vi "DecodeImageArray.vi"(5 "Height":i32, 6 "Pixel Format":T1, 7 "Width":i32, 8 "error in (no error)":errorcluster, 10 "Array":u8[](array[numeric]), 11 "image  in":T2) -> (0 "error out":errorcluster, 3 "image out":T2)   [LabVIEW 2021]
uses:
  <vilib>/vision/Image Controls.llb/IMAQ Image.ctl
  PixelFormat.ctl
  bayer_decode.ctl
panel:
  out "Raw Bytes Per frame":i32
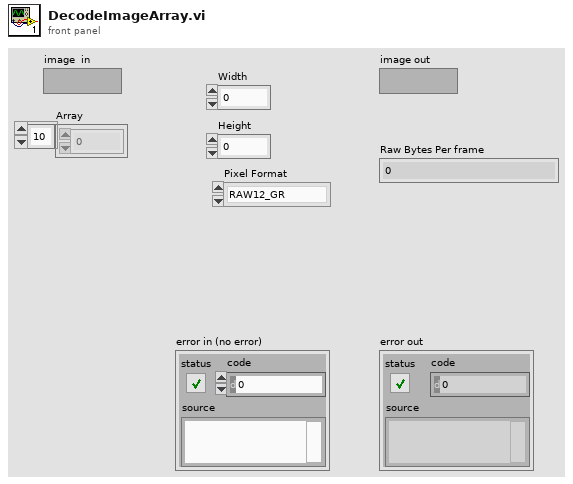
[diagram p1: front panel]
types:
  T1 = typedef "PixelFormat.ctl" = enum16{"RAW12_GR", "YUV422", "RGB888", "RAW8_GR"}
  T2 = typedef "IMAQ Image.ctl" = refnum<image>
  T3 = typedef "Image Type" = u32
  T4 = typedef "bayer_decode.ctl" = enum16{"Bilinear", "VNG"}
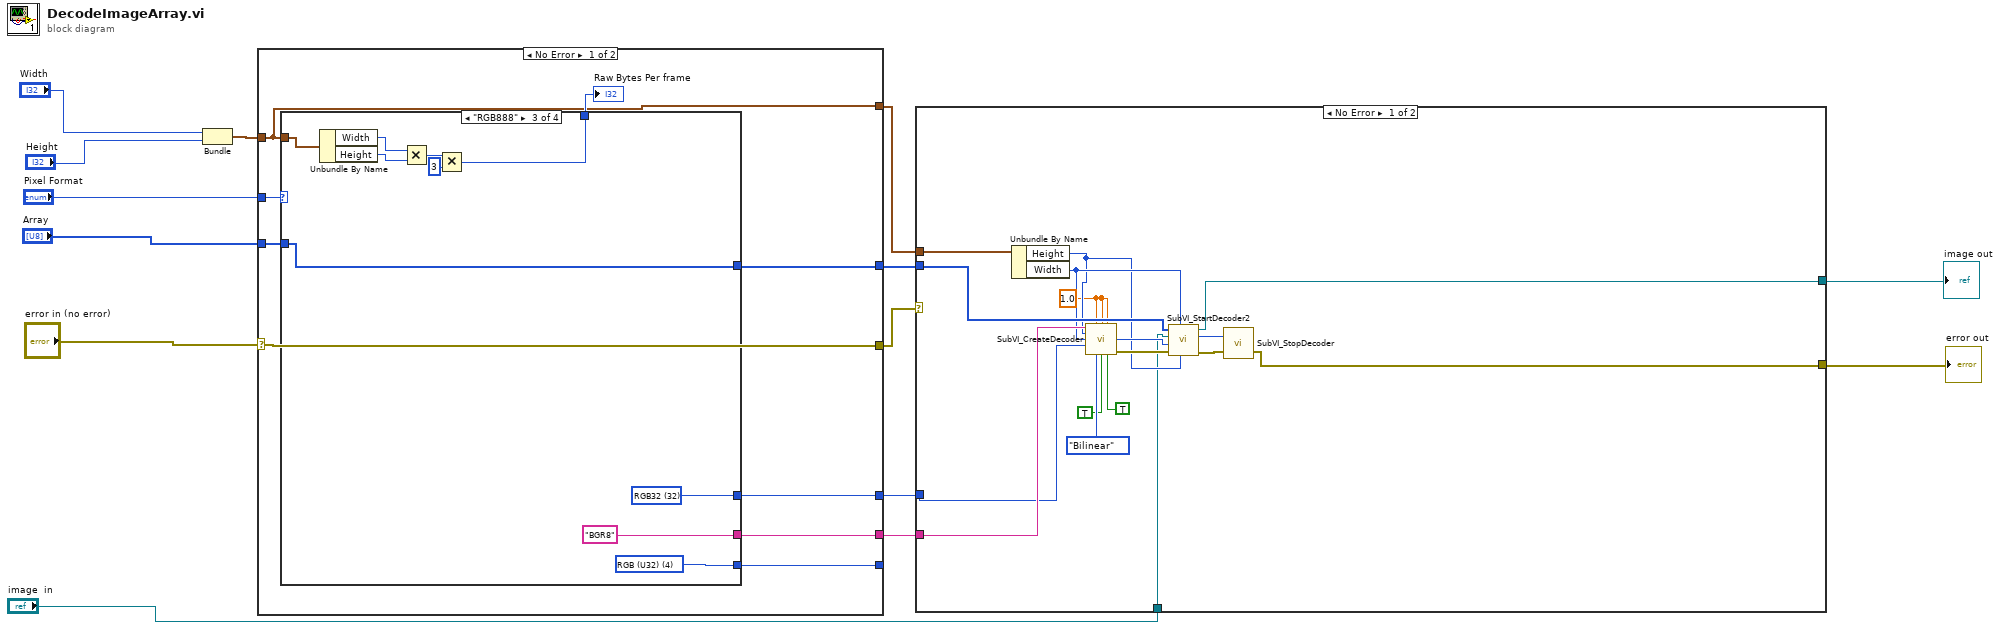
[diagram p0: block diagram]
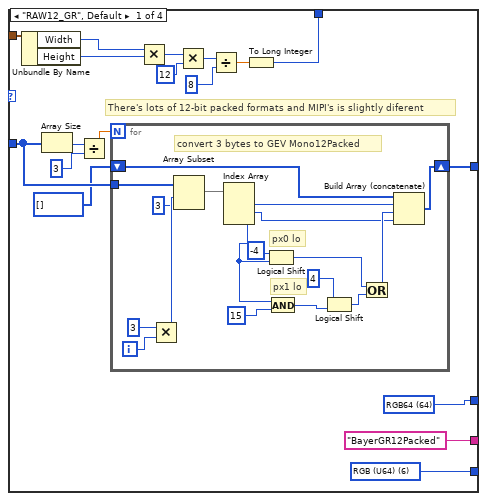
[diagram p2: hidden frame]
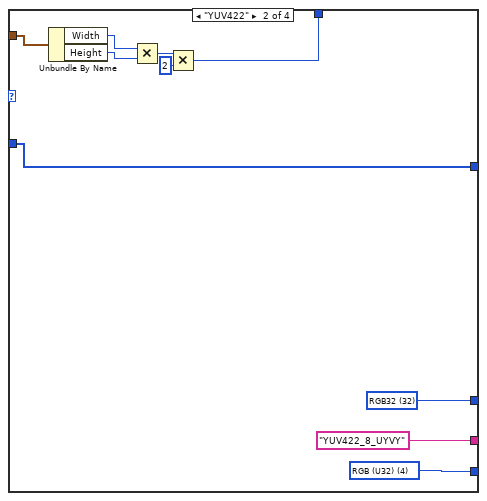
[diagram p3: hidden frame]
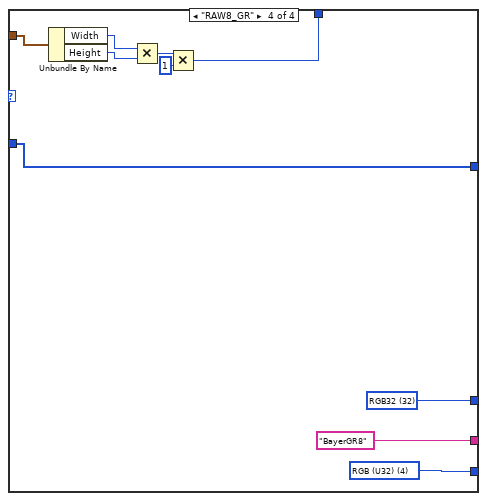
[diagram p4: hidden frame]
diagram:
  n1 = Bundle("Width"="Width", "Height"="Height") -> (w9:cluster{"Width":i32, "Height":i32})  [unwired: 1 in]
  n2 = case shown="No Error" "error in (no error)" {
    selector: "error in (no error)" -> [w18 w90]
    tunnel: "Pixel Format" -> [w23 _]
    tunnel: [w22 _] -> _
    tunnel: "Array" -> [w21 _]
    tunnel: [w19 _] -> w11
    tunnel: [w18 w90] -> w4
    tunnel: [w17 _] -> w5
    tunnel: [w16 _] -> w6
    tunnel: w9 -> [w15 _]
    tunnel: [w15 _] -> w10
    frame No Error {
      n3 = case shown="\"RGB888\"" w23 {
        tunnel: [w36 w67 w77 w87] -> w22
        tunnel: w21 -> [w34 w65 w75 w85]
        tunnel: [w35 w66 w76 w86] -> w20
        tunnel: [w29 w65 w75 w85] -> w19
        tunnel: ["BayerGR12Packed" "YUV422_8_UYVY" "BGR8" "BayerGR8"] -> w17
        tunnel: [w24 w63 w73 w83] -> w16
        tunnel: w15 -> [w27 w62 w72 w82]
        frame "RAW12_GR", Default {
          w24 = u16 64 items=["RGB32"=32, "RGB64"=64] ("Output Bitdepth")
          w36 = T3 6 items=["Grayscale (U8)", "Grayscale (I16)", "Grayscale (SGL)", "Complex (CSG)", "RGB (U32)", "HSL (U32)", "RGB (U64)", "Grayscale (U16)"] ("Image Type")
          # "There's lots of 12-bit packed formats and MIPI's is slightly diferent"
          n4 = Unbundle By Name(w27) -> ("Width"=w26:i32, "Height"=w25:i32)
          n5 = Array Size(array=w34) -> (size(s)=w33:i32)
          n6 = Divide(x=w33, y=3) -> (x/y=w31:dbl)
          n7 = for {
            N: w31 -> [_]
            shift-right: [w42] -> w29
            shift-left: u8[] [] -> [w44]
            tunnel: w34 -> [w59]
            i -> [w58]
            # "convert 3 bytes to GEV Mono12Packed"
            # "px0 lo"
            # "px1 lo"
            n8 = Multiply(x=3, y=w58) -> (x*y=w56:i32)
            n9 = Array Subset(array=w59, index=w56, length=3) -> (w54:u8[])
            n10 = Index Array(array=w54) -> (element #1=w53:u8, element #2=w43:u8, element #3=w51:u8)  [unwired: 3 in]
            n11 = Logical Shift(y=i8 -4 ("x"), x=w51) -> (x << y=w46:u8)
            n12 = And(x=w51, y=u8 15) -> (x .and. y?=w49:u8)
            n13 = Logical Shift(y=i16 4, x=w49) -> (x << y=w47:u8)
            n14 = Or(x=w46, y=w47) -> (x .or. y?=w45:u8)
            n15 = Build Array (concatenate)(w44, w53, w45, w43) -> (w42:u8[])
          }
          n16 = Multiply(x=w26, y=w25) -> (x*y=w41:i32)
          n17 = Multiply(x=w41, y=12) -> (x*y=w39:i32)
          n18 = Divide(x=w39, y=8) -> (x/y=w37:dbl)
          n19 = To Long Integer(number=w37) -> (32bit integer=w35:i32)
        }
        frame "YUV422" {
          w63 = u16 32 items=["RGB32"=32, "RGB64"=64] ("Output Bitdepth")
          w67 = T3 4 items=["Grayscale (U8)", "Grayscale (I16)", "Grayscale (SGL)", "Complex (CSG)", "RGB (U32)", "HSL (U32)", "RGB (U64)", "Grayscale (U16)"] ("Image Type")
          n20 = Unbundle By Name(w62) -> ("Width"=w61:i32, "Height"=w60:i32)
          n21 = Multiply(x=w61, y=w60) -> (x*y=w69:i32)
          n22 = Multiply(x=w69, y=2) -> (x*y=w66:i32)
        }
        frame "RGB888" {
          w73 = u16 32 items=["RGB32"=32, "RGB64"=64] ("Output Bitdepth")
          w77 = T3 4 items=["Grayscale (U8)", "Grayscale (I16)", "Grayscale (SGL)", "Complex (CSG)", "RGB (U32)", "HSL (U32)", "RGB (U64)", "Grayscale (U16)"] ("Image Type")
          n23 = Unbundle By Name(w72) -> ("Width"=w71:i32, "Height"=w70:i32)
          n24 = Multiply(x=w71, y=w70) -> (x*y=w79:i32)
          n25 = Multiply(x=w79, y=3) -> (x*y=w76:i32)
        }
        frame "RAW8_GR" {
          w83 = u16 32 items=["RGB32"=32, "RGB64"=64] ("Output Bitdepth")
          w87 = T3 4 items=["Grayscale (U8)", "Grayscale (I16)", "Grayscale (SGL)", "Complex (CSG)", "RGB (U32)", "HSL (U32)", "RGB (U64)", "Grayscale (U16)"] ("Image Type")
          n26 = Unbundle By Name(w82) -> ("Width"=w81:i32, "Height"=w80:i32)
          n27 = Multiply(x=w81, y=w80) -> (x*y=w89:i32)
          n28 = Multiply(x=w89, y=1) -> (x*y=w86:i32)
        }
      }
      "Raw Bytes Per frame" <- w20
    }
    frame Error {
    }
  }
  n29 = case shown="No Error" w4 {
    selector: w4 -> [_ w108]
    tunnel: w5 -> [w107 _]
    tunnel: w6 -> [w106 _]
    tunnel: w10 -> [w102 _]
    tunnel: w11 -> [w98 _]
    tunnel: [w93 _] -> w12
    tunnel: [w92 w108] -> w13
    tunnel: "image  in" -> [w91 _]
    frame No Error {
      w94 = 1.0 ("redGain")
      n30 = Unbundle By Name(w102) -> ("Height"=w95:i32, "Width"=w97:i32)
      n31 = call "SubVI_CreateDecoder.vi"("pixelFormat"=w107, "redGain"=w94, "greenGain"=w94, "blueGain"=w94, "height"=w95, "width"=w97, "Output Bitdepth"=w106, "Bayer Decode Algorithm"=bayer_decode."Bilinear", "Right Shift Data?"=TRUE, "needsSwap"=TRUE) -> ("decoder"=w99:u64, "error"=w100:errorcluster)  [unwired: 4 in]
      n32 = call "SubVI_StartDecoder2.vi"("height"=w95, "width"=w97, "error in"=w100, "decoder in"=w99, "Destination Image In"=w91, "Source Image In"=w98) -> ("error"=w101:errorcluster, "decoder out"=w96:u64, "Destination Image Out"=w93:T2)  [unwired: 2 in, 1 out]
      n33 = call "SubVI_StopDecoder.vi"("error in"=w101, "decoder in"=w96) -> ("error"=w92:errorcluster)  [unwired: 1 in]
    }
    frame Error {
    }
  }
  "error out" <- w13
  "image out" <- w12
